vi "GlobalBeamDiagnosticSettings.vi"() -> ()   [LabVIEW 2011]
panel:
  out "BeamDiagnosticParameter":i32[](array[numeric])
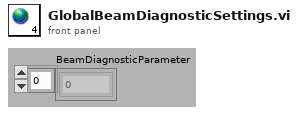
[diagram p1: front panel]
diagram:
